vi "Creat property.vi"(10 "Cluster":T2, 11 "reference":refnum<vi>) -> (1 "Position":T1, 2 "output cluster":T2, 3 "ClusterConstantreference":refnum<vi>)   [LabVIEW 2015]
uses:
  <vilib>/Utility/miscctls.llb/LVPositionTypeDef.ctl
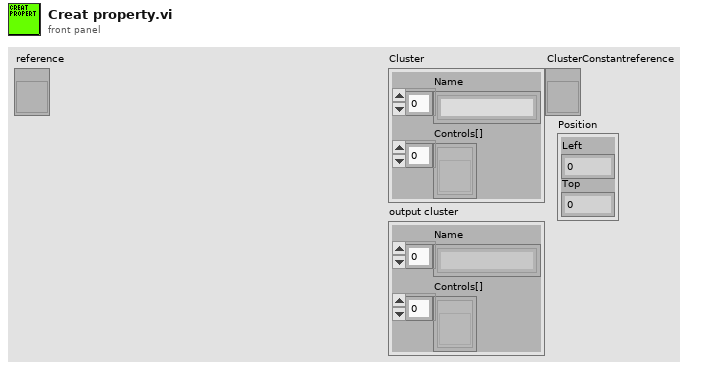
[diagram p1: front panel]
types:
  T1 = typedef "LVPositionTypeDef.ctl" = cluster{"Left":i32, "Top":i32}
  T2 = cluster{"Name":string[], "Controls[]":refnum<vi>[]}
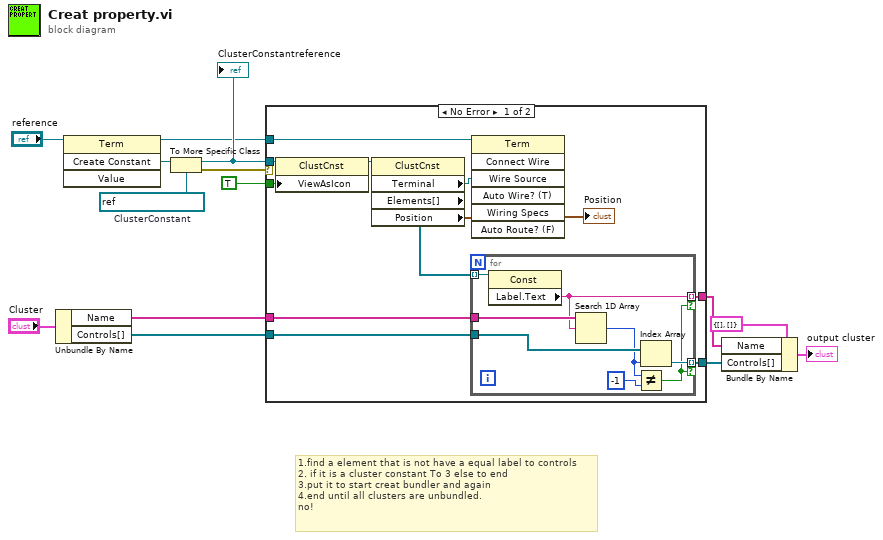
[diagram p0: block diagram]
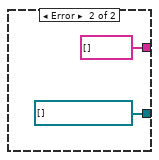
[diagram p2: hidden frame]
diagram:
  w14 = refnum<vi> refnum  # ClusterConstant
  # "1.find a element that is not have a equal label to controls\n2. if it is a cluster constant To 3 else to end \n3.put it to start creat bundler and again\n4.end until all clusters are unbundled.\nno!"
  n1 = Unbundle By Name("Cluster") -> ("Name"=w7:string[], "Controls[]"=w6:refnum<vi>[])
  n2 = invoke class="Term" method="Create Constant"(reference="reference") -> (reference out=w8:refnum<vi>, "Create Constant"=w12:refnum<vi>)  [unwired: 3 in, 2 out]
  n3 = To More Specific Class(target class=w14, reference=w12) -> (specific class reference=w11:refnum<vi>, error out=w13:errorcluster)  [unwired: 1 in]
  "ClusterConstantreference" <- w11
  n4 = case shown="No Error" w13 {
    tunnel: w11 -> [w17 _]
    tunnel: w8 -> [w24 _]
    tunnel: w7 -> [w22 _]
    tunnel: w6 -> [w21 _]
    tunnel: [w20 refnum<vi>[] []] -> w4
    tunnel: [w19 string[] []] -> w5
    tunnel: TRUE -> [w15 _]
    frame No Error {
      n5 = property class="ClustCnst"(reference=w17, "ViewAsIcon"=w15) -> (reference out=w16:refnum<vi>)  [unwired: 1 in, 1 out]
      n6 = property class="ClustCnst"(reference=w16) -> ("Terminal"=w25:refnum<vi>, "Elements[]"=w23:refnum<vi>[], "Position"=→"Position":T1)  [unwired: 1 in, 2 out]
      n7 = for {
        tunnel: w23 -> [w32] mode=indexing
        tunnel: w22 -> [w33]
        tunnel: w21 -> [w31]
        tunnel: [w30] -> w20 mode=indexing if=w26
        tunnel: [w27] -> w19 mode=indexing if=w26
        n8 = property class="Const"(reference=w32) -> ("Label.Text"=w27:string)  [unwired: 1 in, 2 out]
        n9 = Search 1D Array(1D array=w33, element=w27) -> (index of element=w28:i32)  [unwired: 1 in]
        n10 = Not Equal?(x=w28, y=-1 ("x")) -> (x != y?=w26:bool)
        n11 = Index Array(array=w31, index=w28) -> (element=w30:refnum<vi>)
      }
      n12 = invoke class="Term" method="Connect Wire"(reference=w24, "Wire Source"=w25) -> ()  [unwired: 5 in, 7 out]
    }
    frame Error {
    }
  }
  n13 = Bundle By Name(cluster=T2 {"Name"=[], "Controls[]"=[]} ("Cluster"), "Name"=w5, "Controls[]"=w4) -> (→"output cluster":T2)
